vi "Add VI Extension.vi"(10 "VI Name":string) -> (2 "VI Name with .vi":string)   [LabVIEW 2020, in "PropertyBinder.lvlib"]
uses:
  PropertyBinder.lvlib
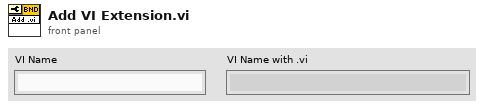
[diagram p1: front panel]
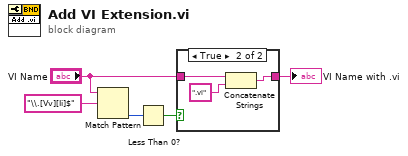
[diagram p0: block diagram]
diagram:
  n1 = Match Pattern(string="VI Name", regular expression="\\.[Vv][Ii]$") -> (offset past match=w4:i32)  [unwired: 1 in, 3 out]
  n2 = Less Than 0?(x=w4) -> (x < 0?=w2:bool)
  n3 = case shown="True" w2 {
    tunnel: "VI Name" -> [w6 w9]
    tunnel: [w6 w7] -> w1
    frame False {
    }
    frame True {
      n4 = Concatenate Strings(w9, ".vi" ("string")) -> (w7:string)
    }
  }
  "VI Name with .vi" <- w1
